vi "AddExperiment.vi"(2 "error in (no error)":errorcluster, 3 "Experiment Name":string, 4 "Visible":bool=TRUE) -> (0 "error out":errorcluster, 1 "Quit ?":bool)   [LabVIEW 2011]
panel:
  in  "MultiCastRemotePort":string
  in  "cwReprate":string
  in  "Experiment Root Path":string
  in  "Multi Cast IP":u16(ring) items=["192.168.10.12", "192.168.10.17", "192.168.10.18", "192.168.10.23", "192.168.10.31", "192.168.10.33", "192.168.10.34", "192.168.10.61", "192.168.10.64", "192.168.10.63", "192.168.10.65", "192.168.10.68", "192.168.10.69", "192.168.10.71", "192.168.10.72", "192.168.10.91", "192.168.10.92", "192.168.10.93", "192.168.10.94", "192.168.10.99", "192.168.10.110", "192.168.10.114", "192.168.10.150", "192.168.10.36", "192.168.10.153", "192.168.10.156", "192.168.10.157", "192.168.10.182", "192.168.10.183", "192.168.10.184", "192.168.10.186", "192.168.10.187", "192.168.10.189", "192.168.10.213", "192.168.12.76", "192.168.12.195", "192.168.10.73", "192.168.10.75", "192.168.10.21", "192.168.10.88", "192.168.10.113", "192.168.10.115", "192.168.10.116", "192.168.10.122", "192.168.10.123", "192.168.10.125", "192.168.10.126", "192.168.10.127", "192.168.10.128", "192.168.10.124", "192.168.10.11", "192.168.10.152", "192.168.10.155", "192.168.10.35", "192.168.10.60", "192.168.10.67", "192.168.10.95", "192.168.0.19", "192.168.0.19", "192.168.0.19"]
  in  "Quit":bool
  in  "Create Experiment":bool
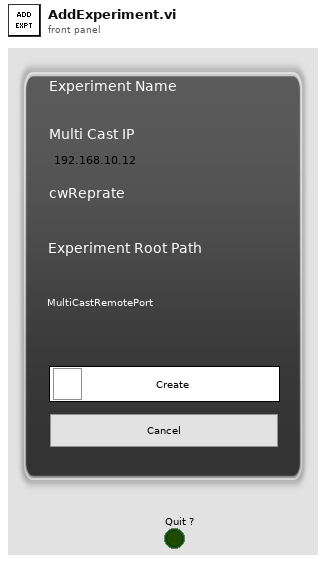
[diagram p1: front panel]
types:
  T1 = typedef "mysql_authentication.ctl" = cluster{"User":string, "Password":string, "Database":string}
  T2 = cluster{"Port":u16, "IP Address":string, "Authentication":T1}
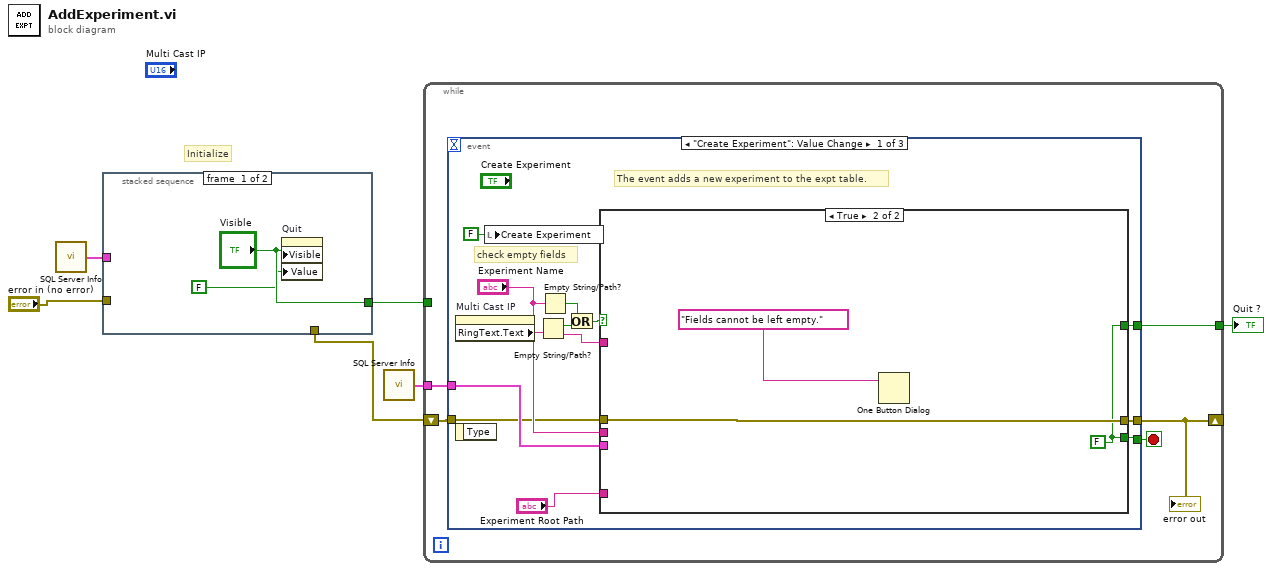
[diagram p0: block diagram]
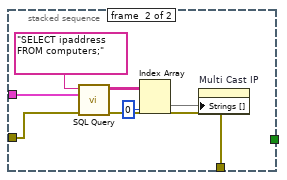
[diagram p2: hidden frame]
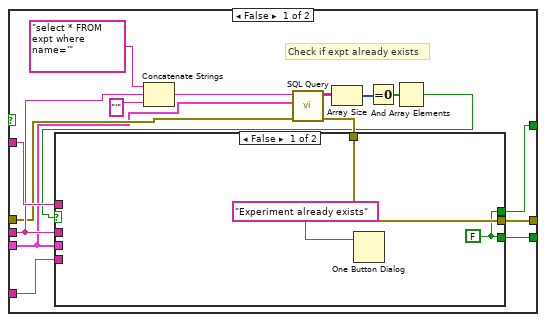
[diagram p3: hidden frame]
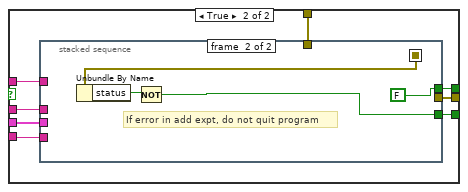
[diagram p4: hidden frame]
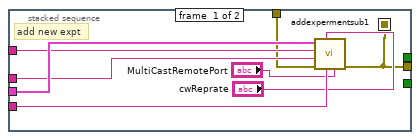
[diagram p5: hidden frame]
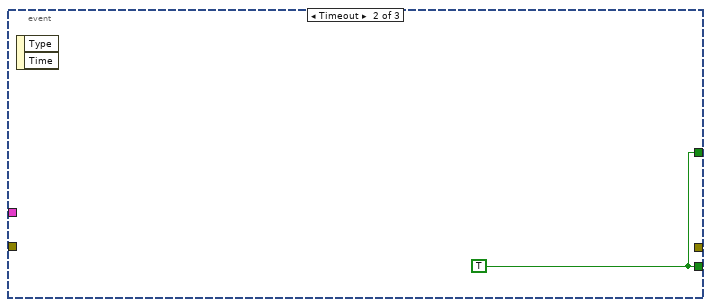
[diagram p6: hidden frame]
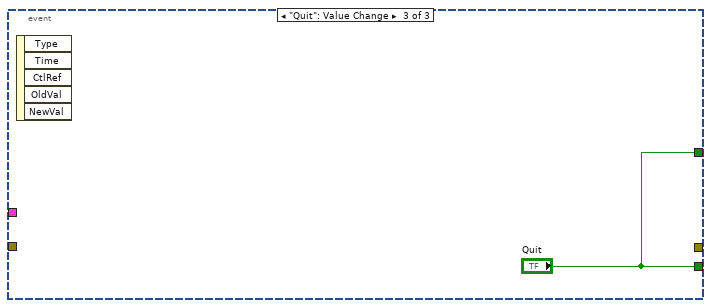
[diagram p7: hidden frame]
diagram:
  # "Initialize"
  n1 = call "SQL Server Info.vi"() -> ("SQL Server Info"=w4:T2)
  n2 = stacked-sequence {
    tunnel: ["Visible" _] -> w5
    tunnel: w4 -> [_ w11]
    tunnel: "error in (no error)" -> [_ w10]
    tunnel: [_ w9] -> w2
    frame #0 {
      n3 = property on="Quit" class="Bool (strict)"("Visible"="Visible", "Value"=FALSE ("Quit")) -> ()  [unwired: 2 in, 2 out]
    }
    frame #1 {
      n4 = call "SQL Query.vi"("error in (no error)"=w10, "SQL Server Info"=w11, "Query"="SELECT ipaddress  FROM computers;") -> ("error out"=w9:errorcluster, "data"=w13:string[][])  [unwired: 7 in]
      n5 = Index Array(array=w13, index (col)=0 ("disabled index (col)")) -> (element=w15:string[])  [unwired: 1 in]
      n6 = property on="Multi Cast IP" class="Ring (strict)"("Strings []"=w15) -> ()  [unwired: 2 in, 2 out]
    }
  }
  n7 = call "SQL Server Info.vi"() -> ("SQL Server Info"=w6:T2)
  n8 = while {
    tunnel: w6 -> [w20]
    tunnel: w5 -> [_]
    shift-right: [w18] -> _
    shift-left: w2 -> [w17]
    tunnel: [w16] -> w1
    stop <- w19 stop-if-true
    n9 = event shown="[0] \"Create Experiment\": Value Change" {
      selector: _ -> [_ _ _]
      dyn-events: _ -> [_ _ _]
      timeout: _ -> [_ _ _]
      tunnel: [w22 w75 "Quit"] -> w19
      tunnel: w20 -> [w32 _ _]
      tunnel: [w27 _ _] -> w18
      tunnel: w17 -> [w26 _ _]
      tunnel: [w21 w75 "Quit"] -> w16
      event "Create Experiment": Value Change {
        # "check empty fields"
        # "The event adds a new experiment to the expt table."
        n10 = property on="Multi Cast IP" class="Ring (strict)"() -> ("RingText.Text"=w25:string)  [unwired: 2 in, 2 out]
        n11 = event-data() -> ()  [unwired: 1 in, 1 out]
        n12 = local write "Create Experiment"(FALSE ("Create Experiment")) -> ()
        n13 = Empty String/Path?(string/path=w25) -> (empty?=w30:bool)
        n14 = Empty String/Path?(string/path="Experiment Name") -> (empty?=w29:bool)
        n15 = Or(x=w29, y=w30) -> (x .or. y?=w28:bool)
        n16 = case shown="True" w28 {
          tunnel: w32 -> [w36 _]
          tunnel: "Experiment Name" -> [w41 _]
          tunnel: w25 -> [w48 _]
          tunnel: [w39 w73] -> w27
          tunnel: w26 -> [w38 w73]
          tunnel: "Experiment Root Path" -> [w35 _]
          tunnel: [w34 w72] -> w22
          tunnel: [w33 w72] -> w21
          frame False {
            # "Check if expt already exists"
            n17 = Concatenate Strings("select * FROM expt where name='" ("Query"), w41, "'" ("string")) -> (w45:string)
            n18 = call "SQL Query.vi"("error in (no error)"=w38, "SQL Server Info"=w36, "Query"=w45) -> ("error out"=w40:errorcluster, "data"=w44:string[][])  [unwired: 7 in]
            n19 = Array Size(array=w44) -> (size(s)=w43:i32[])
            n20 = Equal To 0?(x=w43) -> (x = 0?=w42:bool[])
            n21 = And Array Elements(Boolean array=w42) -> (logical AND=w37:bool)
            n22 = case shown="False" w37 {
              tunnel: w36 -> [_ w59]
              tunnel: w48 -> [_ w58]
              tunnel: w41 -> [_ w57]
              tunnel: w40 -> [w51 w56]
              tunnel: [w51 w55] -> w39
              tunnel: w35 -> [_ w54]
              tunnel: [w49 w53] -> w34
              tunnel: [w49 w52] -> w33
              frame False {
                w49 = FALSE
                n23 = One Button Dialog(message="Experiment already exists") -> ()  [unwired: 1 in, 1 out]
              }
              frame True {
                n24 = stacked-sequence {
                  seq-local: [w60 _] -> [_ w71]
                  tunnel: w59 -> [w67 _]
                  tunnel: w58 -> [w66 _]
                  tunnel: w57 -> [w65 _]
                  tunnel: w56 -> [w64 _]
                  tunnel: [w60 _] -> w55
                  tunnel: w54 -> [w63 _]
                  tunnel: [_ w69] -> w53
                  tunnel: [_ FALSE] -> w52
                  frame #0 {
                    # "add new expt"
                    n25 = call "addexpermentsub1.vi"("MultiCastRemotePort"="MultiCastRemotePort", "Experiment Root Path"=w63, "cwReprate"="cwReprate", "error in (no error)"=w64, "Experiment Name"=w65, "Multi Cast IP"=w66, "SQL Server Info"=w67) -> ("error IO"=w60:errorcluster)  [unwired: 4 in]
                  }
                  frame #1 {
                    # "If error in add expt, do not quit program"
                    n26 = Unbundle By Name(w71) -> ("status"=w70:bool)
                    n27 = Not(x=w70) -> (.not. x?=w69:bool)
                  }
                }
              }
            }
          }
          frame True {
            w72 = FALSE
            n28 = One Button Dialog(message="Fields cannot be left empty.") -> ()  [unwired: 1 in, 1 out]
          }
        }
      }
      event Timeout {
        w75 = TRUE
        n29 = event-data() -> ()  [unwired: 1 in, 2 out]
      }
      event "Quit": Value Change {
        n30 = event-data() -> ()  [unwired: 1 in, 5 out]
      }
    }
    "error out" <- w18
  }
  "Quit ?" <- w1
